vi "Initialize Imaging Control.vi"(8 "error in":errorcluster, 11 "IMG_SRC in":refnum<class "IMG_SRC.lvclass">) -> (0 "error out":errorcluster, 3 "IMG_SRC out":refnum<class "IMG_SRC.lvclass">)   [LabVIEW 2018, in "IMG_SRC.lvlib" / "IMG_SRC.lvclass"]
uses:
  IMG_SRC.lvclass
  IMG_SRC.lvclass/IMG_SRC.ctl
panel:
  in  "ICImagingControl":refnum<k7>(container)
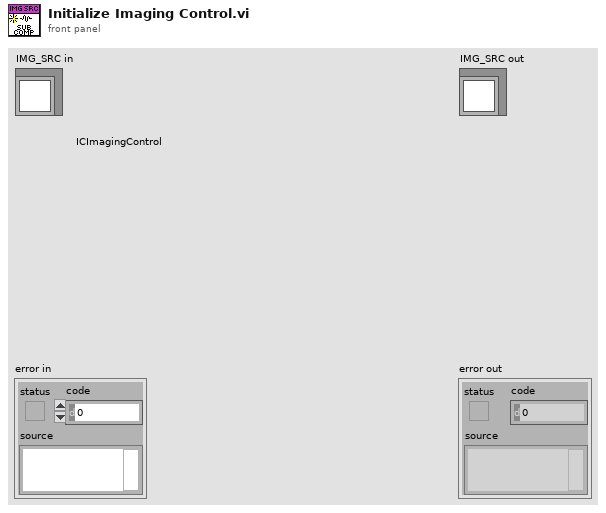
[diagram p1: front panel]
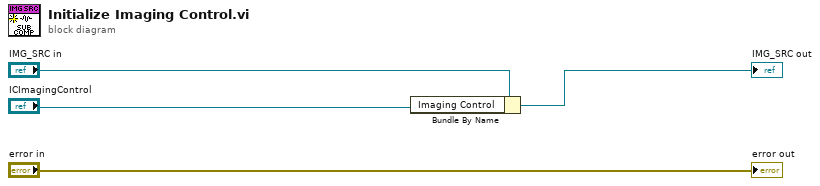
[diagram p0: block diagram]
diagram:
  n1 = Bundle By Name(cluster="IMG_SRC in", "Imaging Control"="ICImagingControl") -> (→"IMG_SRC out":refnum<class "IMG_SRC.lvclass">)
  "error out" <- "error in"
